vi "32 and 12 pulses TX 8spc_ver2.vi"(7 "reset system clock":bool, 8 "referenses":T1={"clock x2"="IO Socket\\Data Clock 2x", "Memory In"="pulse on memory", "Memory In 2"="pulse on memory", "Memory In 3"="pulse on memory", "Memory In 4"="pulse on memory", "Memory In 5"="pulse on memory", "Memory In 6"="pulse on memory", "Memory In 7"="pulse on memory", "Memory In 8"="pulse on memory", "Memory In 9"="pulse on memory", "Memory In 10"="pulse on memory", "Memory In 11"="pulse on memory", "Memory In 12"="pulse on memory"}, 9 "IQ_run":bool=TRUE, 10 "PDW input Valid":bool, 11 "array PDW":u64[](array[numeric])=[0, 0, 0, 0]) -> (0 "trig out":bool, 1 "pulse TX status":T2, 2 "output valid":bool, 3 "IQ out":T3[](array[typedef]), 4 "ready for input":bool)   [LabVIEW 2021]
uses:
  <instrlib>/_niInstr/DSP/v1/Shared/Public/IQ Data.ctl
  pulse_tx_vis/CTL/mode_type.ctl
  <instrlib>/_niInstr/Basic Elements/v1/FPGA/Private/Count Up U64.vi
  <instrlib>/_niInstr/Basic Elements/v1/FPGA/Private/Count Up U32.vi
  <instrlib>/_niInstr/Basic Elements/v1/FPGA/niInstr Basic Elements v1 FPGA.lvlib
  <instrlib>/_niInstr/DSP/v1/Shared/niInstr DSP v1 Shared.lvlib
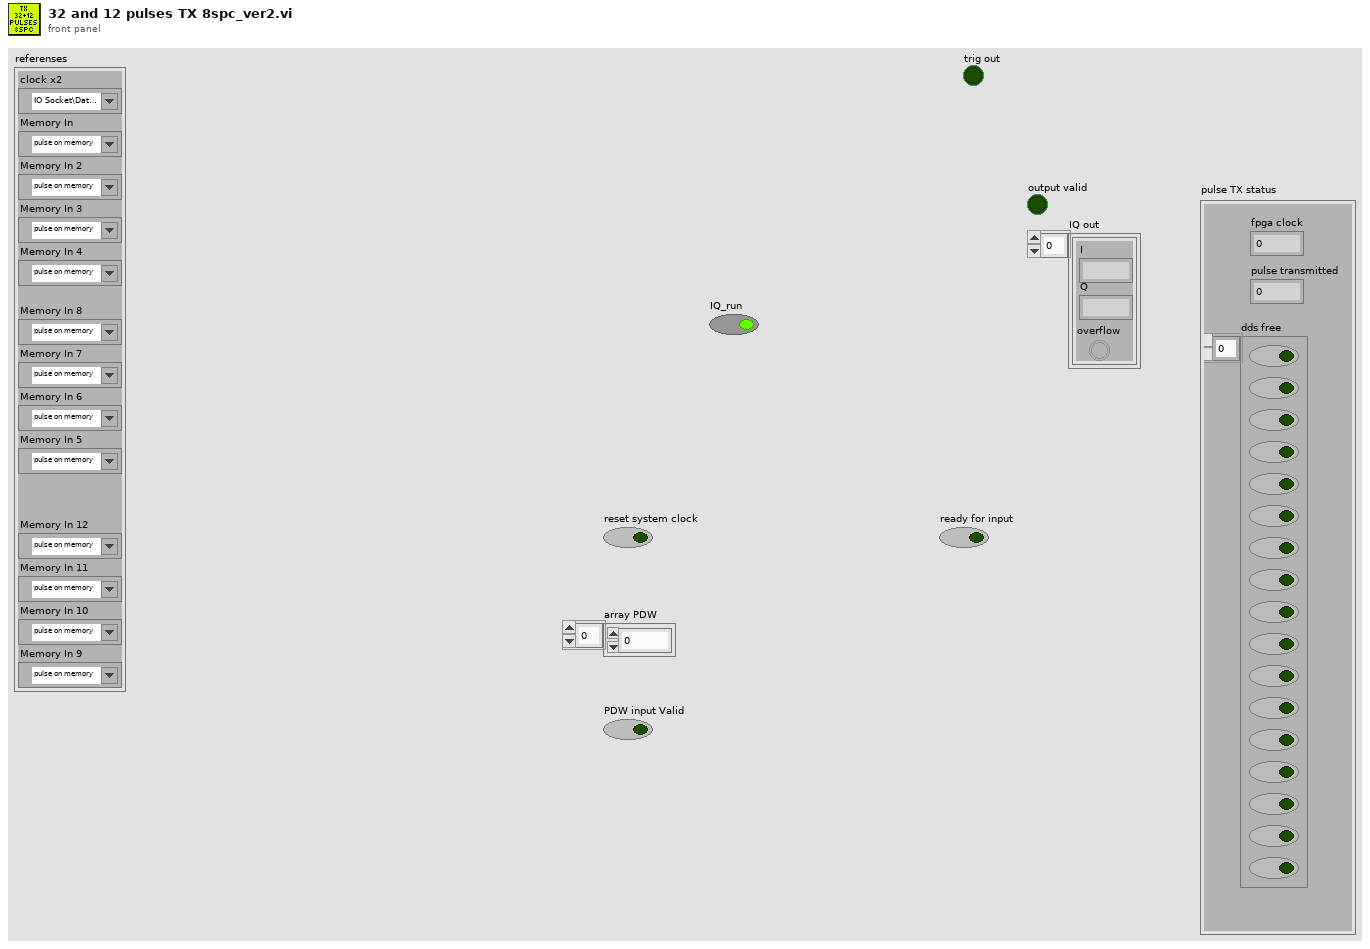
[diagram p1: front panel]
types:
  T1 = cluster{"clock x2":refnum<k21>, "Memory In":refnum<k21>, "Memory In 2":refnum<k21>, "Memory In 3":refnum<k21>, "Memory In 4":refnum<k21>, "Memory In 5":refnum<k21>, "Memory In 6":refnum<k21>, "Memory In 7":refnum<k21>, "Memory In 8":refnum<k21>, "Memory In 9":refnum<k21>, "Memory In 10":refnum<k21>, "Memory In 11":refnum<k21>, "Memory In 12":refnum<k21>}
  T2 = cluster{"fpga clock":u64, "pulse transmitted":u32, "dds free":bool[]}
  T3 = typedef "niInstr DSP v1 Shared.lvlib/IQ Data.ctl" = cluster{"I":fxp<+/-,18,1>, "Q":fxp<+/-,18,1>, "overflow":bool}
  T4 = cluster{"clock x2":refnum<k21>, "Memory In":refnum<k21>, "Memory In 2":refnum<k21>, "Memory In 3":refnum<k21>, "Memory In 4":refnum<k21>}
  T5 = typedef "mode_type.ctl" = enum8{"CW", "from memory 1", "NC - cw", "LFM", "BPSK", "QPSK"}
  T6 = typedef "pdw.ctl" = cluster{"PW":u32, "frequency shift":fxp<+/-,48,0>, "amp":fxp<+/-,18,1>, "mode type":T5, "mode depth":u32, "mode filter":u8, "phase shift":fxp<+/-,16,1>, "pulse shape filter":u8}
  T7 = cluster{"I":fxp<+/-,18,1>, "Q":fxp<+/-,18,1>, "overflow":bool}[]
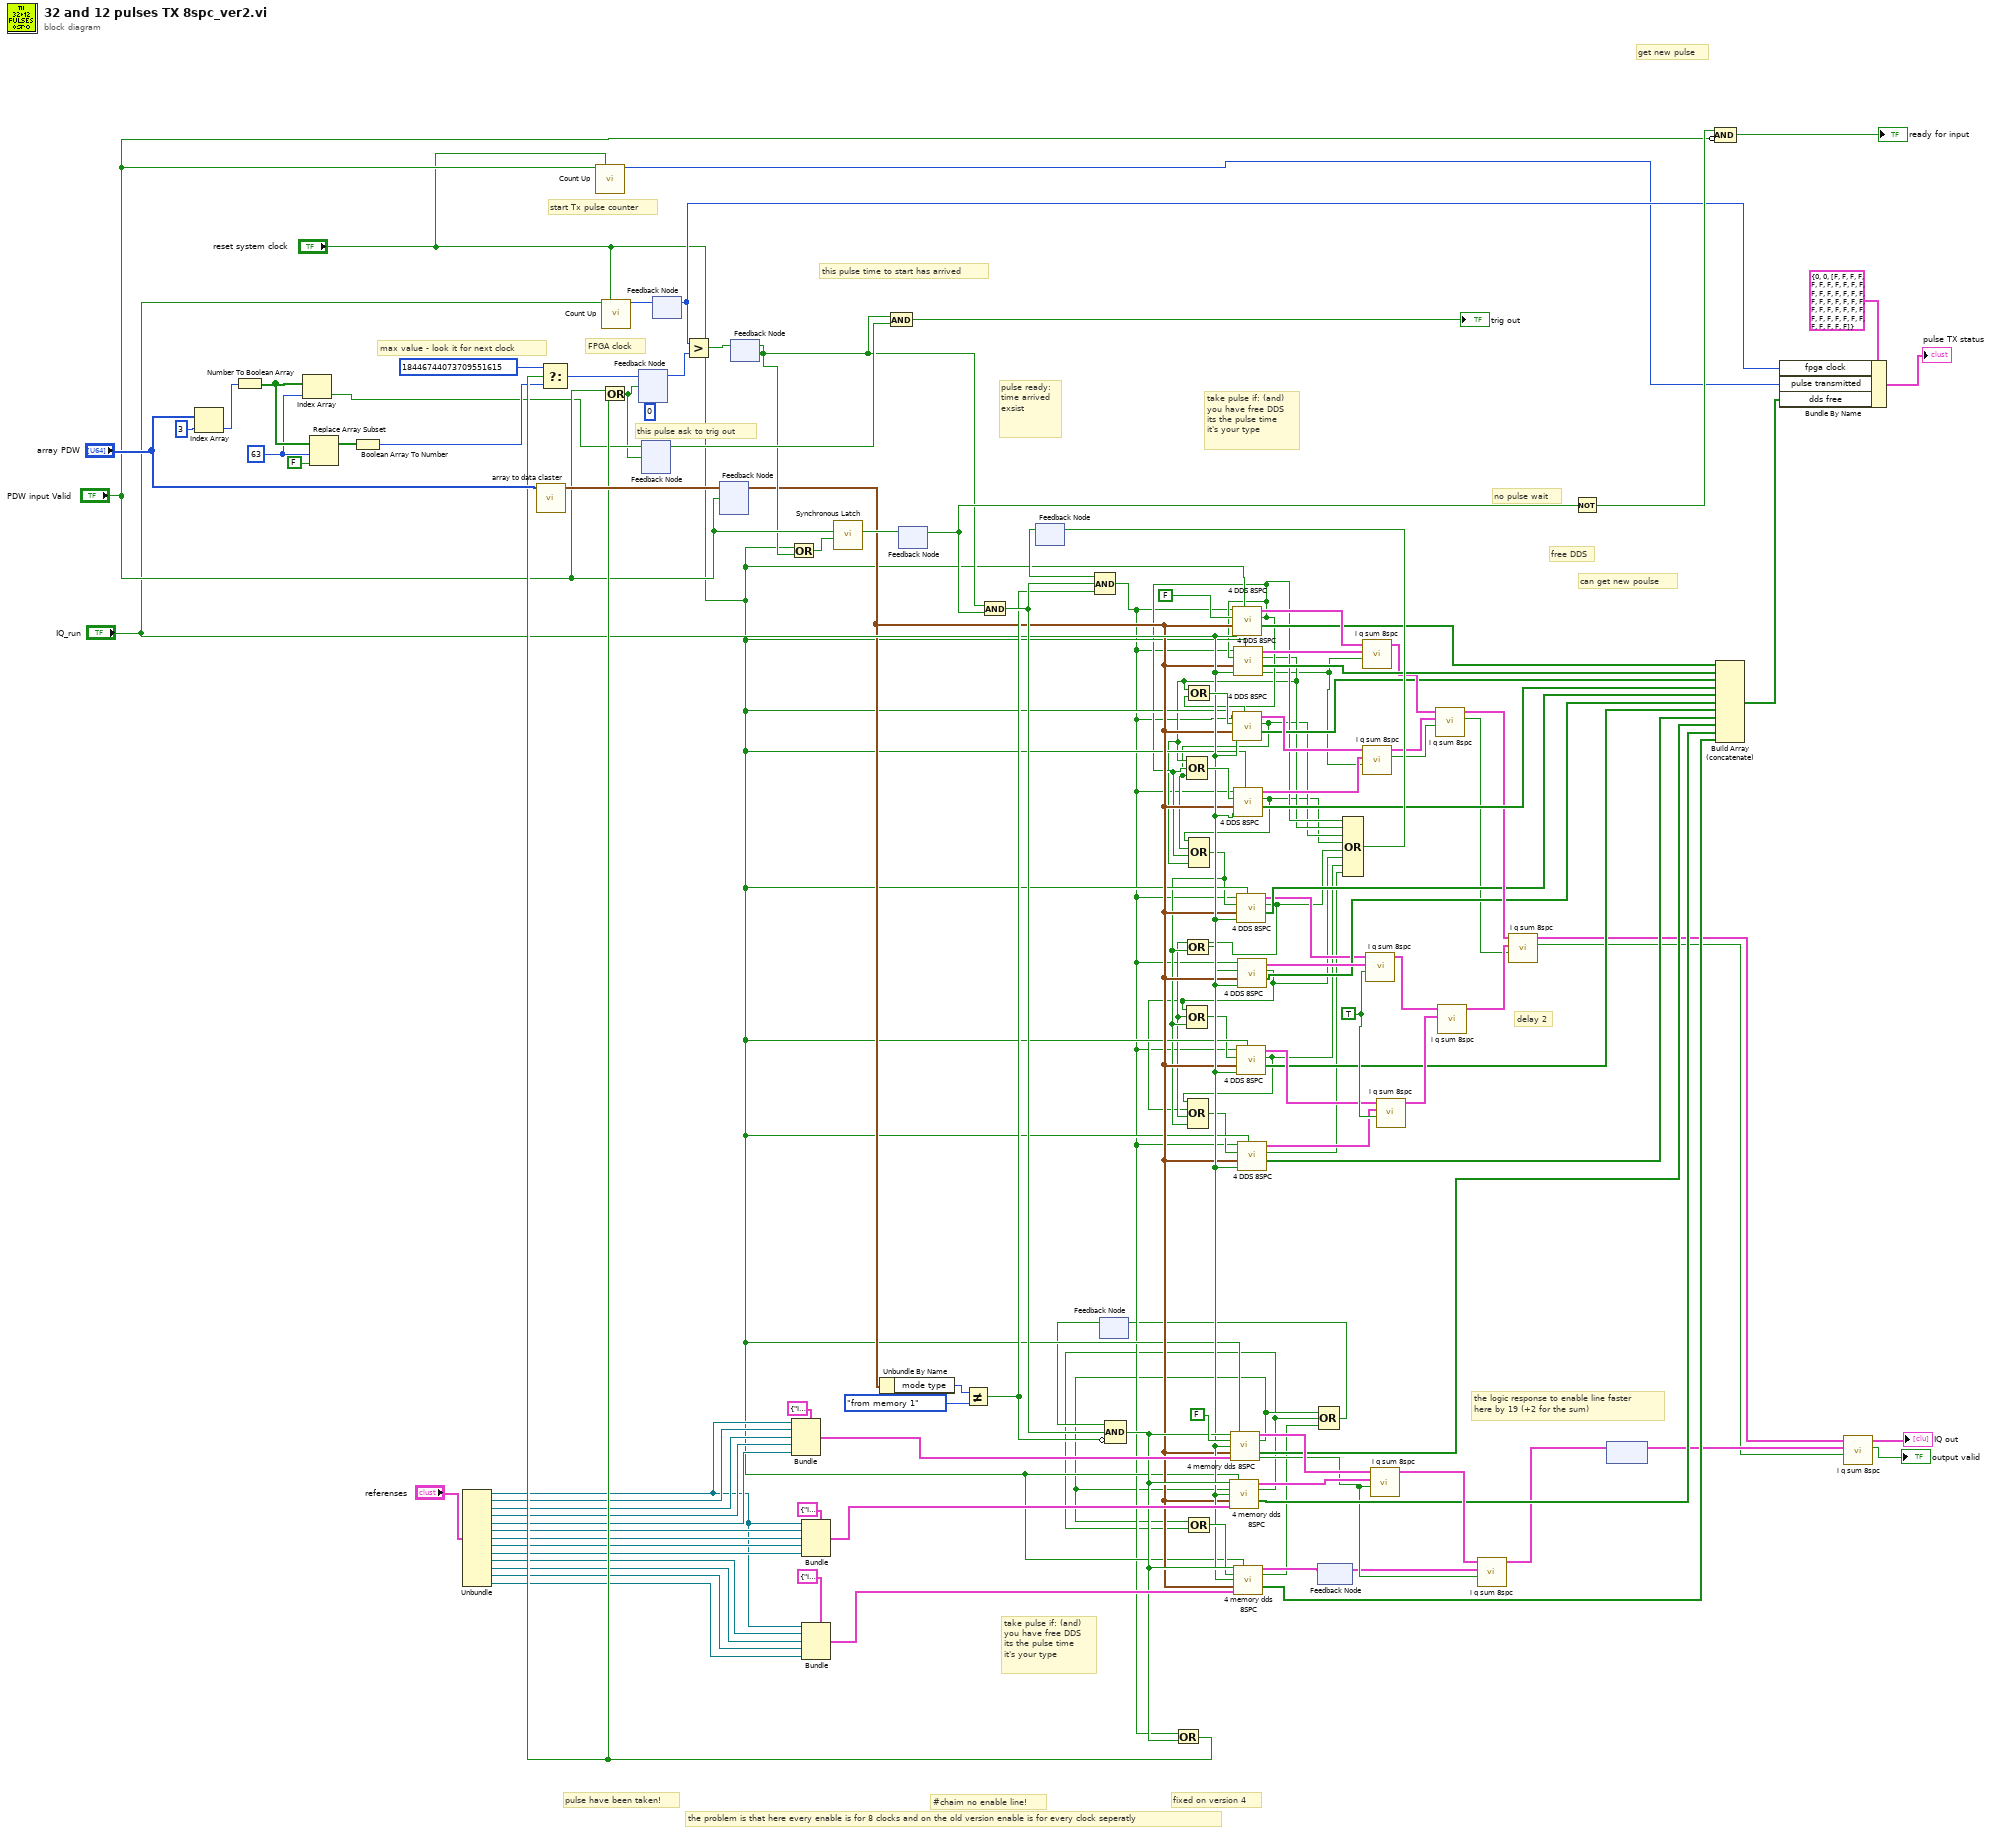
[diagram p0: block diagram]
diagram:
  w44 = TRUE ("input valid")
  w89 = 63 ("index")
  # "the logic response to enable line faster\nhere by 19 (+2 for the sum)"
  # "delay 2"
  # "fixed on version 4"
  # "this pulse ask to trig out"
  # "pulse ready:\ntime arrived\nexsist"
  # "take pulse if: (and)\nyou have free DDS\nits the pulse time\nit's your type"
  # "take pulse if: (and)\nyou have free DDS\nits the pulse time\nit's your type"
  # "pulse have been taken!"
  # "the problem is that here every enable is for 8 clocks and on the old version enable is for every clock seperatly"
  # "#chaim no enable line!"
  # "start Tx pulse counter"
  # "FPGA clock"
  # "this pulse time to start has arrived"
  # "max value - look it for next clock"
  # "get new pulse"
  # "can get new poulse"
  # "no pulse wait"
  # "free DDS"
  n1 = Index Array(array="array PDW", index=3) -> (element=w91:u64)
  n2 = Number To Boolean Array(number=w91) -> (Boolean array=w90:bool[])
  n3 = Index Array(array=w90, index=w89) -> (element=w85:bool)
  n4 = Replace Array Subset(array=w90, new element=FALSE ("new element/subarray"), index=w89) -> (w87:bool[])
  n5 = Boolean Array To Number(Boolean array=w87) -> (number=w86:u64)
  n6 = Unbundle("referenses") -> ("clock x2"=w55:refnum<k21>, "Memory In"=w67:refnum<k21>, "Memory In 2"=w66:refnum<k21>, "Memory In 3"=w65:refnum<k21>, "Memory In 4"=w64:refnum<k21>, "Memory In 5"=w63:refnum<k21>, "Memory In 6"=w62:refnum<k21>, "Memory In 7"=w61:refnum<k21>, "Memory In 8"=w60:refnum<k21>, "Memory In 9"=w54:refnum<k21>, "Memory In 10"=w53:refnum<k21>, "Memory In 11"=w52:refnum<k21>, "Memory In 12"=w51:refnum<k21>)
  n7 = call "array to data claster.vi"("Array"="array PDW") -> ("Cluster"=w108:T6)  [unwired: 10 in]
  n8 = call-poly <instrlib>:"Count Up.vi"("increment"="PDW input Valid", "reset"="reset system clock") -> ("count out"=w112:u32)  [unwired: 13 in]
  n9 = call-poly <instrlib>:"Count Up.vi"("increment"="IQ_run", "reset"="reset system clock") -> ("count out"=w122:u64)  [unwired: 13 in]
  n10 = feedback #1(u64 0 ("U64")) -> (w116:u64)
  n11 = feedback #2() -> (w83:bool)  [unwired: 1 in]
  n12 = feedback #3() -> (w113:u64)  [unwired: 1 in]
  n13 = feedback-in #3(w122) -> ()
  n14 = Greater?(x=w113, y=w116) -> (0:w126:bool)
  n15 = feedback #4() -> (w31:T6)  [unwired: 1 in]
  n16 = feedback-in #4(w108, "PDW input Valid") -> ()
  n17 = feedback #5() -> (w82:bool)  [unwired: 1 in]
  n18 = feedback-in #5(w126) -> ()
  n19 = Or(x="reset system clock", y=w82) -> (x .or. y?=w95:bool)
  n20 = Bundle(cluster=T4 {"clock x2"="IO Socket\\Data Clock 2x", "Memory In"="pulse on memory", "Memory In 2"="pulse on memory", "Memory In 3"="pulse on memory", "Memory In 4"="pulse on memory"} ("referenses"), "clock x2"=w55, "Memory In"=w67, "Memory In 2"=w66, "Memory In 3"=w65, "Memory In 4"=w64) -> (w59:T4)
  n21 = Bundle(cluster=T4 {"clock x2"="IO Socket\\Data Clock 2x", "Memory In"="pulse on memory", "Memory In 2"="pulse on memory", "Memory In 3"="pulse on memory", "Memory In 4"="pulse on memory"} ("referenses"), "clock x2"=w55, "Memory In"=w63, "Memory In 2"=w62, "Memory In 3"=w61, "Memory In 4"=w60) -> (w58:T4)
  n22 = Bundle(cluster=T4 {"clock x2"="IO Socket\\Data Clock 2x", "Memory In"="pulse on memory", "Memory In 2"="pulse on memory", "Memory In 3"="pulse on memory", "Memory In 4"="pulse on memory"} ("referenses"), "clock x2"=w55, "Memory In"=w54, "Memory In 2"=w53, "Memory In 3"=w52, "Memory In 4"=w51) -> (w50:T4)
  n23 = call <instrlib>:"Synchronous Latch.vi"("clear"=w95, "set"="PDW input Valid") -> ("out"=w93:bool)  [unwired: 9 in]
  n24 = Unbundle By Name(w31) -> ("mode type"=w110:T5)
  n25 = And(x=w82, y=w83) -> (x .and. y?=→"trig out":bool)
  n26 = feedback #6() -> (w92:bool)  [unwired: 1 in]
  n27 = feedback-in #6(w93) -> ()
  n28 = Not Equal?(x=w110, y=mode_type."from memory 1") -> (x != y?=w104:bool)
  n29 = And(x=w82, y=w92) -> (x .and. y?=w105:bool)
  n30 = feedback #7() -> (w101:bool)  [unwired: 1 in]
  n31 = Compound Arithmetic op=AND(w101, w105, w104) -> (w8:bool)
  n32 = feedback #8() -> (w3:bool)  [unwired: 1 in]
  n33 = Compound Arithmetic op=AND(w3, w105, invert w104) -> (w49:bool)
  n34 = Or(x=w8, y=w49) -> (x .or. y?=w102:bool)
  n35 = Select(t=u64 18446744073709551615, s=w102, f=w86) -> (s? t:f=w120:u64)
  n36 = Or(x="PDW input Valid", y=w102) -> (x .or. y?=w84:bool)
  n37 = feedback-in #1(w120, w84) -> ()
  n38 = feedback-in #2(w85, w84) -> ()
  n39 = call "4 memory dds 8SPC.vi"("new PDW in"=w49, "stop this pulse"="reset system clock", "free DDS before me?"=FALSE, "run"="IQ_run", "pdw in"=w31, "referenses"=w59) -> ("IQ out"=w76:T3[], "have free DDS"=w2:bool, "state of every DDS"=w47:bool[], "output valid"=w23:bool)  [unwired: 6 in]
  n40 = call "4 memory dds 8SPC.vi"("new PDW in"=w49, "stop this pulse"="reset system clock", "free DDS before me?"=w2, "run"="IQ_run", "pdw in"=w31, "referenses"=w58) -> ("IQ out"=w75:T3[], "have free DDS"=w1:bool, "state of every DDS"=w46:bool[])  [unwired: 6 in, 1 out]
  n41 = Compound Arithmetic op=OR(w2, w1) -> (w48:bool)
  n42 = call "4 DDS 8SPC.vi"("clear DDS"="reset system clock", "input valid"="IQ_run", "pdw in"=w31, "free DDS before me?"=FALSE, "new PDW in"=w8) -> ("state of every DDS"=w97:bool[], "have free DDS"=w29:bool, "IQ out"=w100:T3[])  [unwired: 3 in, 1 out]
  n43 = call "4 DDS 8SPC.vi"("clear DDS"="reset system clock", "input valid"="IQ_run", "pdw in"=w31, "free DDS before me?"=w29, "new PDW in"=w8) -> ("output valid"=w24:bool, "state of every DDS"=w96:bool[], "have free DDS"=w28:bool, "IQ out"=w99:T3[])  [unwired: 3 in]
  n44 = Compound Arithmetic op=OR(w28, w29) -> (w73:bool)
  n45 = call "4 DDS 8SPC.vi"("clear DDS"="reset system clock", "input valid"="IQ_run", "pdw in"=w31, "free DDS before me?"=w73, "new PDW in"=w8) -> ("state of every DDS"=w71:bool[], "have free DDS"=w15:bool, "IQ out"=w80:T3[])  [unwired: 3 in, 1 out]
  n46 = Compound Arithmetic op=OR(w28, w29, w15) -> (w74:bool)
  n47 = call "4 DDS 8SPC.vi"("clear DDS"="reset system clock", "input valid"="IQ_run", "pdw in"=w31, "free DDS before me?"=w74, "new PDW in"=w8) -> ("state of every DDS"=w72:bool[], "have free DDS"=w14:bool, "IQ out"=w79:T3[])  [unwired: 3 in, 1 out]
  n48 = Compound Arithmetic op=OR(w14, w15, w29, w28) -> (w25:bool)
  n49 = call "4 memory dds 8SPC.vi"("new PDW in"=w49, "stop this pulse"="reset system clock", "free DDS before me?"=w48, "run"="IQ_run", "pdw in"=w31, "referenses"=w50) -> ("IQ out"=w7:T3[], "have free DDS"=w5:bool, "state of every DDS"=w45:bool[])  [unwired: 6 in, 1 out]
  n50 = call "4 DDS 8SPC.vi"("clear DDS"="reset system clock", "input valid"="IQ_run", "pdw in"=w31, "free DDS before me?"=w25, "new PDW in"=w8) -> ("state of every DDS"=w36:bool[], "have free DDS"=w13:bool, "IQ out"=w22:T3[])  [unwired: 3 in, 1 out]
  n51 = Compound Arithmetic op=OR(w13, w25) -> (w9:bool)
  n52 = call "4 DDS 8SPC.vi"("input valid"="IQ_run", "pdw in"=w31, "free DDS before me?"=w9, "new PDW in"=w8) -> ("state of every DDS"=w35:bool[], "have free DDS"=w12:bool, "IQ out"=w39:T3[])  [unwired: 4 in, 1 out]
  n53 = Compound Arithmetic op=OR(w12, w13, w25) -> (w27:bool)
  n54 = call "4 DDS 8SPC.vi"("clear DDS"="reset system clock", "input valid"="IQ_run", "pdw in"=w31, "free DDS before me?"=w27, "new PDW in"=w8) -> ("state of every DDS"=w34:bool[], "have free DDS"=w11:bool, "IQ out"=w40:T3[])  [unwired: 3 in, 1 out]
  n55 = Compound Arithmetic op=OR(w11, w12, w13, w25) -> (w26:bool)
  n56 = call "4 DDS 8SPC.vi"("clear DDS"="reset system clock", "input valid"="IQ_run", "pdw in"=w31, "free DDS before me?"=w26, "new PDW in"=w8) -> ("state of every DDS"=w33:bool[], "have free DDS"=w10:bool, "IQ out"=w41:T3[])  [unwired: 3 in, 1 out]
  n57 = feedback #9() -> (w6:T3[])  [unwired: 1 in]
  n58 = feedback-in #9(w7) -> ()
  n59 = Compound Arithmetic op=OR(w2, w1, w5) -> (w4:bool)
  n60 = feedback-in #8(w4) -> ()
  n61 = Compound Arithmetic op=OR(w29, w28, w15, w14, w13, w12, w11, w10) -> (w98:bool)
  n62 = feedback-in #7(w98) -> ()
  n63 = call "i q sum 8spc.vi"("input valid"=w24, "IQ in 2"=w99, "IQ in"=w100) -> ("IQ out"=w77:T7)  [unwired: 7 in, 1 out]
  n64 = call "i q sum 8spc.vi"("input valid"=w24, "IQ in 2"=w79, "IQ in"=w80) -> ("output valid"=w19:bool, "IQ out"=w78:T7)  [unwired: 7 in]
  n65 = call "i q sum 8spc.vi"("input valid"=w44, "IQ in 2"=w39, "IQ in"=w22) -> ("IQ out"=w43:T7)  [unwired: 7 in, 1 out]
  n66 = call "i q sum 8spc.vi"("input valid"=w23, "IQ in 2"=w75, "IQ in"=w76) -> ("IQ out"=w57:T7)  [unwired: 7 in, 1 out]
  n67 = call "i q sum 8spc.vi"("input valid"=w44, "IQ in 2"=w41, "IQ in"=w40) -> ("IQ out"=w42:T7)  [unwired: 7 in, 1 out]
  n68 = call "i q sum 8spc.vi"("input valid"=w19, "IQ in 2"=w78, "IQ in"=w77) -> ("output valid"=w20:bool, "IQ out"=w38:T7)  [unwired: 7 in]
  n69 = call "i q sum 8spc.vi"("IQ in 2"=w42, "IQ in"=w43) -> ("IQ out"=w37:T7)  [unwired: 8 in, 1 out]
  n70 = call "i q sum 8spc.vi"("input valid"=w23, "IQ in 2"=w6, "IQ in"=w57) -> ("IQ out"=w18:T7)  [unwired: 7 in, 1 out]
  n71 = call "i q sum 8spc.vi"("input valid"=w20, "IQ in 2"=w37, "IQ in"=w38) -> ("output valid"=w16:bool, "IQ out"=w21:T7)  [unwired: 7 in]
  n72 = Not(x=w92) -> (.not. x?=w117:bool)
  n73 = feedback #10() -> (w17:T7)  [unwired: 1 in]
  n74 = feedback-in #10(w18) -> ()
  n75 = Compound Arithmetic op=AND(w117, invert "PDW input Valid") -> (→"ready for input":bool)
  n76 = Build Array (concatenate)(w97, w96, w71, w72, w36, w35, w34, w33, w47, w46, w45) -> (w111:bool[])
  n77 = Bundle By Name(cluster=T2 {"fpga clock"=0, "pulse transmitted"=0, "dds free"=[FALSE, FALSE, FALSE, FALSE, FALSE, FALSE, FALSE, FALSE, FALSE, FALSE, FALSE, FALSE, FALSE, FALSE, FALSE, FALSE, FALSE, FALSE, FALSE, FALSE, FALSE, FALSE, FALSE, FALSE, FALSE, FALSE, FALSE, FALSE, FALSE, FALSE, FALSE, FALSE, FALSE, FALSE, FALSE, FALSE, FALSE, FALSE, FALSE, FALSE, FALSE, FALSE, FALSE, FALSE]} ("pulse TX status"), "fpga clock"=w113, "pulse transmitted"=w112, "dds free"=w111) -> (→"pulse TX status":T2)
  n78 = call "i q sum 8spc.vi"("input valid"=w16, "IQ in 2"=w17, "IQ in"=w21) -> ("output valid"=→"output valid":bool, "IQ out"=→"IQ out":T7)  [unwired: 7 in]
